vi "URG-04LX-UG01 Close.vi"(8 "error in":errorcluster, 11 "VISA Refnum in":refnum<visa-resource-name>) -> (0 "error out":errorcluster)   [LabVIEW 2018]
doc: "Ends the Hokuyo URG-04LX-UG01 session."
uses:
  Type Definitions/Hokuyo Command Parameter.ctl
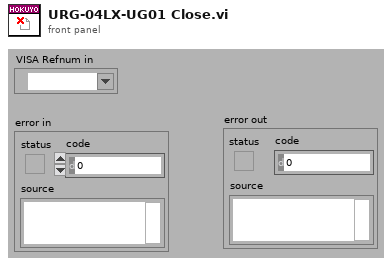
[diagram p1: front panel]
types:
  T1 = typedef "Hokuyo Command Parameter.ctl" = cluster{"Device Command":string, "String Characters":string}
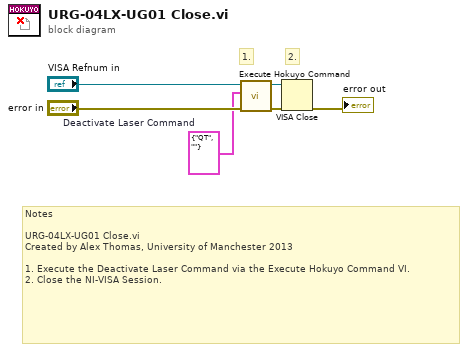
[diagram p0: block diagram]
diagram:
  w4 = T1 {"Device Command"="QT", "String Characters"=""}  # Deactivate Laser Command
  # "2."
  # "1."
  # "Notes\n\nURG-04LX-UG01 Close.vi\nCreated by Alex Thomas, University of Manchester 2013\n\n1. Execute the Deactivate Laser Command via the Execute Hokuyo Command VI.\n2. Close the NI-VISA Session."
  n1 = call "Execute Hokuyo Command.vi"("error in (no error)"="error in", "Hokuyo Command Parameter"=w4, "VISA Refnum in"="VISA Refnum in") -> ("error out"=w3:errorcluster, "VISA Refnum out"=w2:refnum<visa-resource-name>)  [unwired: 6 in, 1 out]
  n2 = VISA Close(VISA resource name=w2, error in (no error)=w3) -> (error out=→"error out":errorcluster)
